vi "mapping.vi"(8 "spin":dbl(slide) scale=-1.0..1.0, 10 "x":dbl(slide) scale=-1.0..1.0, 11 "y":dbl(slide) scale=-1.0..1.0) -> ()   [LabVIEW 2023]
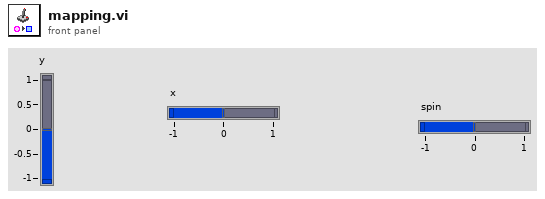
[diagram p1: front panel]
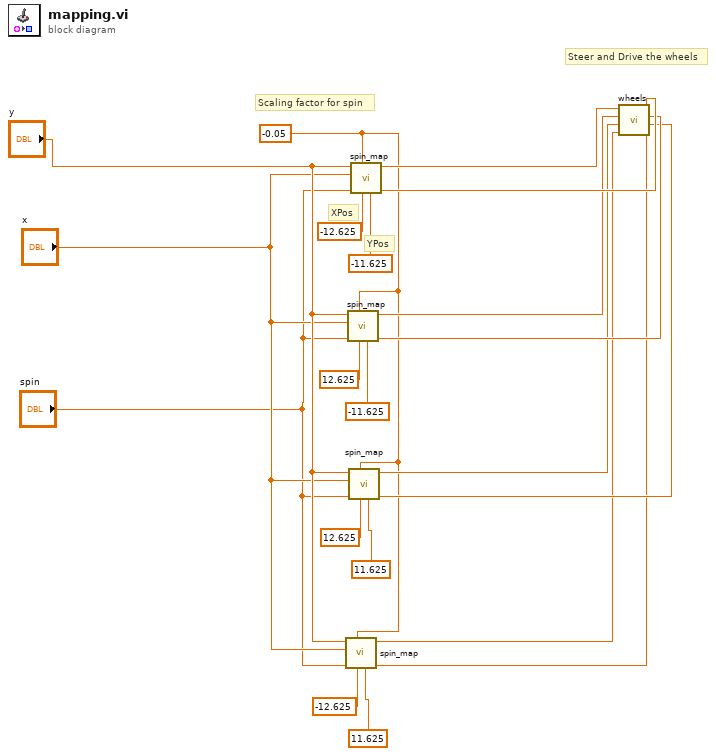
[diagram p0: block diagram]
diagram:
  w1 = -0.05
  # "Steer and Drive the wheels"
  # "YPos"
  # "XPos"
  # "Scaling factor for spin"
  n1 = call "spin_map.vi"("pos_y"=11.625, "pos_x"=-12.625, "scale"=w1, "spin"="spin", "x"="x", "y"="y") -> ("mag"=w2:dbl, "angle"=w3:dbl)  [unwired: 4 in]
  n2 = call "spin_map.vi"("pos_y"=-11.625, "pos_x"=12.625, "scale"=w1, "spin"="spin", "x"="x", "y"="y") -> ("mag"=w13:dbl, "angle"=w14:dbl)  [unwired: 4 in]
  n3 = call "spin_map.vi"("pos_y"=11.625, "pos_x"=12.625, "scale"=w1, "spin"="spin", "x"="x", "y"="y") -> ("mag"=w9:dbl, "angle"=w10:dbl)  [unwired: 4 in]
  n4 = call "spin_map.vi"("pos_y"=-11.625, "pos_x"=-12.625, "scale"=w1, "spin"="spin", "x"="x", "y"="y") -> ("mag"=w19:dbl, "angle"=w20:dbl)  [unwired: 4 in]
  n5 = call "wheels.vi"("Speed 4"=w2, "Speed 3"=w9, "Speed 2"=w13, "Speed 1"=w19, "Steer 4"=w3, "Steer 3"=w10, "Steer 2"=w14, "Steer 1"=w20) -> ()  [unwired: 4 in]
